vi "insertNewScriptEvent.vi"(6 "delayAll":bool=TRUE, 7 "selectedIndex":i32, 8 "error in (no error)":errorcluster, 9 "index":i32=-1, 10 "ScriptEvent":refnum<class "ScriptEvent.lvclass">, 11 "ScriptEventList in":refnum<class "ScriptEventList.lvclass">) -> (0 "error out":errorcluster, 3 "ScriptEventList out":refnum<class "ScriptEventList.lvclass">)   [LabVIEW 2011, in "Tools.lvlib" / "Scripting.lvlib" / "ScriptEventList.lvclass"]
uses:
  ScriptEventList.lvclass
  ScriptEvent.lvclass
  ScriptEventList.lvclass/ScriptEventList.ctl
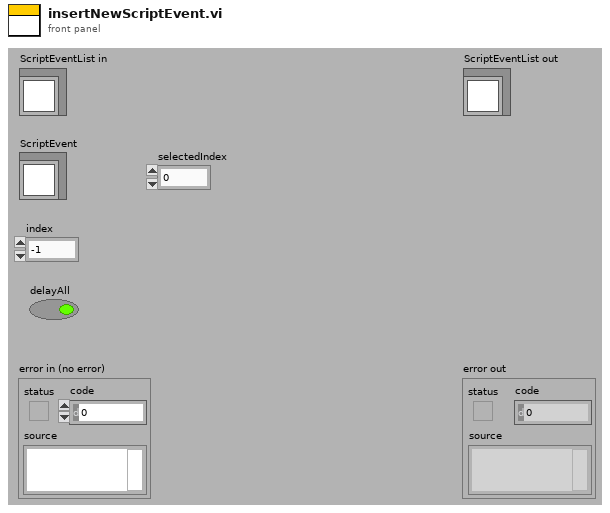
[diagram p1: front panel]
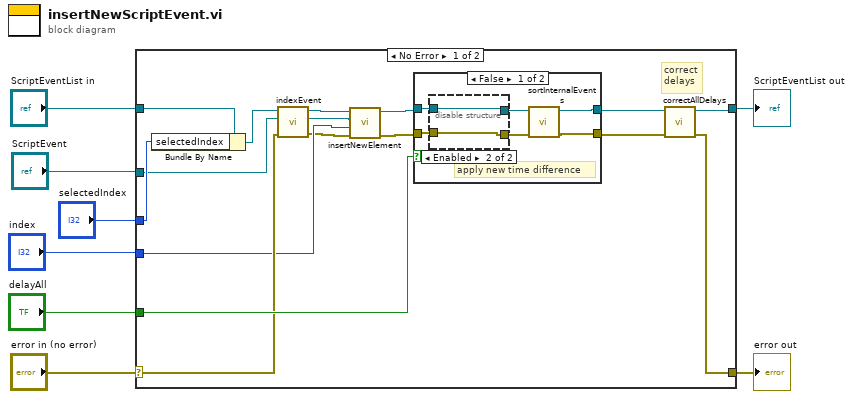
[diagram p0: block diagram]
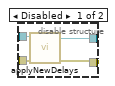
[diagram p2: hidden frame]
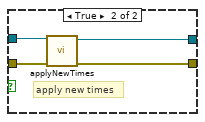
[diagram p3: hidden frame]
diagram:
  n1 = case shown="No Error" "error in (no error)" {
    selector: "error in (no error)" -> [w20 w42]
    tunnel: [w18 w42] -> w7
    tunnel: [w17 w41] -> w5
    tunnel: "ScriptEventList in" -> [w23 w41]
    tunnel: "ScriptEvent" -> [w21 _]
    tunnel: "delayAll" -> [w24 _]
    tunnel: "index" -> [w13 _]
    tunnel: "selectedIndex" -> [w22 _]
    frame No Error {
      # "correct\ndelays"
      n2 = Bundle By Name(cluster=w23, "selectedIndex"=w22) -> (w19:refnum<class "ScriptEventList.lvclass">)
      n3 = call "indexEvent.vi"("error in (no error)"=w20, "ScriptEvent"=w21, "ScriptEventList in"=w19) -> ("error out"=w12:errorcluster, "ScriptEvent out"=w14:refnum<class "ScriptEvent.lvclass">, "ScriptEventList out"=w15:refnum<class "ScriptEventList.lvclass">)  [unwired: 5 in, 1 out]
      n4 = call "insertNewElement.vi"("error in (no error)"=w12, "index"=w13, "ScriptEvent"=w14, "ScriptEventList in"=w15) -> ("error out"=w11:errorcluster, "ScriptEventList out"=w16:refnum<class "ScriptEventList.lvclass">)  [unwired: 6 in]
      n5 = case shown="False" w24 {
        tunnel: w16 -> [w30 w40]
        tunnel: w11 -> [w29 w39]
        tunnel: [w27 w38] -> w10
        tunnel: [w26 w37] -> w9
        frame False {
          # "apply new time difference"
          n6 = disable-structure shown="Enabled" {
            disable-tunnel: w30 -> [w34 w36]
            disable-tunnel: w29 -> [w33 w35]
            disable-tunnel: [w32 w36] -> w28
            disable-tunnel: [w31 w35] -> w25
            frame Disabled {
              n7 = call "applyNewDelays.vi"("error in (no error)"=w33, "ScriptEventList in"=w34) -> ("error out"=w31:errorcluster, "ScriptEventList out"=w32:refnum<class "ScriptEventList.lvclass">)  [unwired: 8 in]
            }
            frame Enabled {
            }
          }
          n8 = call "sortInternalEvents.vi"("error in (no error)"=w25, "ScriptEventList in"=w28) -> ("error out"=w26:errorcluster, "ScriptEventList out"=w27:refnum<class "ScriptEventList.lvclass">)  [unwired: 8 in]
        }
        frame True {
          # "apply new times"
          n9 = call "applyNewTimes.vi"("error in (no error)"=w39, "ScriptEventList in"=w40) -> ("error out"=w37:errorcluster, "ScriptEventList out"=w38:refnum<class "ScriptEventList.lvclass">)  [unwired: 8 in]
        }
      }
      n10 = call "correctAllDelays.vi"("error in (no error)"=w9, "ScriptEventList in"=w10) -> ("error out"=w18:errorcluster, "ScriptEventList out"=w17:refnum<class "ScriptEventList.lvclass">)  [unwired: 8 in]
    }
    frame Error {
    }
  }
  "error out" <- w7
  "ScriptEventList out" <- w5
